vi "ASrreglo0dispINIC.vi"(9 "Y":i32, 10 "X":i32) -> (2 "output array":dbl[][](array[numeric]))   [LabVIEW 2016]
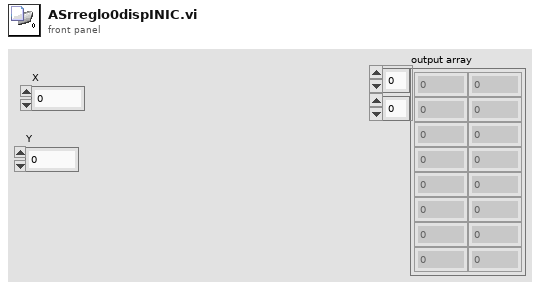
[diagram p1: front panel]
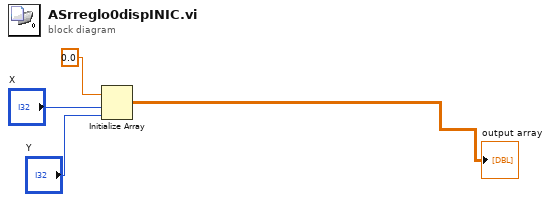
[diagram p0: block diagram]
diagram:
  n1 = Initialize Array(0.0 ("element"), "X", "Y") -> (→"output array":dbl[][])
